vi "Create 3D Shapes.vi"(8 "error in (no error)":errorcluster, 11 "Frame Grabber Data In":T1={"Camera Session"="", "Frame"=refnum, "AVI Refnum"=refnum, "Codecs"=[], "Frame number"=0, "Tracking File Refnum"=refnum, "Tick Count"=0, "Probe Object"=refnum, "Playback Probe Data"=[], "Rigid Body"={"Position"={"x (mm)"=0.0, "y (mm)"=0.0, "z (mm)"=0.0}, "Orientation"={"Pitch (rad)"=0.0, "Yaw (rad)"=0.0, "Roll (rad)"=0.0}, "Quaternion"={"qx"=0.0, "qy"=0.0, "qz"=0.0, "qw"=0.0}, "Tracked?"=FALSE}, "Total no frames playback"=0, "Video FPS"=0.0, "Camera connected?"=FALSE, "Scene"=refnum, "Cropped Frame"=refnum, "Tracker FPS"=0.0, "Crop ROI"=[], "Presentation Values"=[], "Elapsed time (ms)"=0, "Camera frames playback"=0, "Refnums"={"Live Refnum"=refnum, "Record Refnum"=refnum, "Recording Settings Refnum"=refnum, "Playback Refnum"=refnum, "Frame Slider Refnum"=refnum, "Pause Refnum"=refnum, "Home Refnum"=refnum, "Crop Refnum"=refnum, "Clear Crop Refnum"=refnum, "stop refnum"=refnum, "Playback Rate Refnum"=refnum, "Operator Settings Refnums"=refnum, "Presentation Refnum"=refnum, "Gestation Refnum"=refnum, "Crop Time Frame Slider Refnum"=refnum, "Cancel Save Refnum"=refnum, "Reverse Playback Refnum"=refnum, "Connection Settings Refnum"=refnum}, "Dimensions"={"Probe Dimensions"={"Probe Width"=0.0, "Probe Depth"=1.0, "Probe Height"=0.0}, "Room Dimensions"={"Room Width"=0.0, "Room Depth"=0.0, "Room Height"=0.0}}, "Playback Data As Strings"=[], "Cropped Tracking File Refnum"=refnum, "Cropped AVI Refnum"=refnum, "Header"=[], "Total euclidian distance"=0.0, "Annotation File Path"=path "", "Playback File Path"=path ""}) -> (0 "error out":errorcluster={"status"=TRUE, "code"=1088, "source"="Property Node (arg 2) in NI_3D Picture Control.lvlib:Create Box.vi->Create 3D Shapes.vi->Init Frame Grabber.vi->Main.vi"}, 3 "Frame Grabber Data Out":T1={"Camera Session"="", "Frame"=refnum, "AVI Refnum"=refnum, "Codecs"=[], "Frame number"=0, "Tracking File Refnum"=refnum, "Tick Count"=0, "Probe Object"=refnum, "Playback Probe Data"=[], "Rigid Body"={"Position"={"x (mm)"=0.0, "y (mm)"=0.0, "z (mm)"=0.0}, "Orientation"={"Pitch (rad)"=0.0, "Yaw (rad)"=0.0, "Roll (rad)"=0.0}, "Quaternion"={"qx"=0.0, "qy"=0.0, "qz"=0.0, "qw"=0.0}, "Tracked?"=FALSE}, "Total no frames playback"=0, "Video FPS"=0.0, "Camera connected?"=FALSE, "Scene"=refnum, "Cropped Frame"=refnum, "Tracker FPS"=0.0, "Crop ROI"=[], "Presentation Values"=[], "Elapsed time (ms)"=0, "Camera frames playback"=0, "Refnums"={"Live Refnum"=refnum, "Record Refnum"=refnum, "Recording Settings Refnum"=refnum, "Playback Refnum"=refnum, "Frame Slider Refnum"=refnum, "Pause Refnum"=refnum, "Home Refnum"=refnum, "Crop Refnum"=refnum, "Clear Crop Refnum"=refnum, "stop refnum"=refnum, "Playback Rate Refnum"=refnum, "Operator Settings Refnums"=refnum, "Presentation Refnum"=refnum, "Gestation Refnum"=refnum, "Crop Time Frame Slider Refnum"=refnum, "Cancel Save Refnum"=refnum, "Reverse Playback Refnum"=refnum, "Connection Settings Refnum"=refnum}, "Dimensions"={"Probe Dimensions"={"Probe Width"=0.0, "Probe Depth"=1.0, "Probe Height"=0.0}, "Room Dimensions"={"Room Width"=0.0, "Room Depth"=0.0, "Room Height"=0.0}}, "Playback Data As Strings"=[], "Cropped Tracking File Refnum"=refnum, "Cropped AVI Refnum"=refnum, "Header"=[], "Total euclidian distance"=0.0, "Annotation File Path"=path "", "Playback File Path"=path ""})   [LabVIEW 2017]
uses:
  Controls/Frame Grabber Data.ctl
  <vilib>/userdefined/High Color/IMAQdx.ctl
  <vilib>/vision/Image Controls.llb/IMAQ Image.ctl
  <vilib>/vision/Avi.llb/IMAQ AVI2 Refnum.ctl
  Controls/Rigid Body Info.ctl
  Controls/Position.ctl
  Controls/Orientation.ctl
  Controls/Refnums.ctl
  Controls/Recording Settings.ctl
  Controls/Operator Settings.ctl
  Controls/Operator.ctl
  Controls/Connection Settings.ctl
  Controls/Tracker Type.ctl
  Controls/COM Port.ctl
  Controls/Dimensions.ctl
  Controls/Room Dimensions.ctl
  <vilib>/picture/3D Picture Control/Object/Create Object (name).vi
  <vilib>/picture/3D Picture Control/Object/Create Object (drawable).vi
  <vilib>/picture/3D Picture Control/Object/Add Object (no reference).vi
  <vilib>/picture/3D Picture Control/Object/Add Object (reference).vi
  <vilib>/picture/3D Picture Control/NI_3D Picture Control.lvlib
panel:
  out "Probe Object":refnum<vi>
  out "Scene":refnum<vi>(3d-picture)
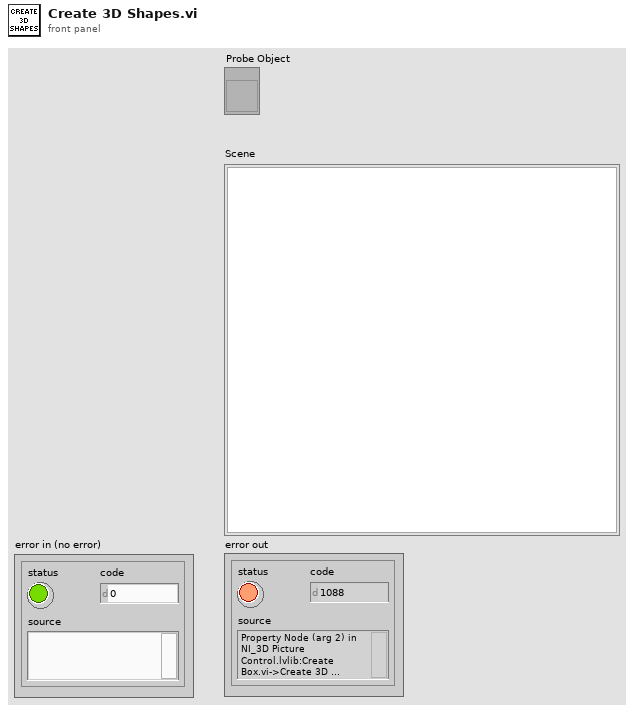
[diagram p1: front panel]
types:
  T1 = typedef "Frame Grabber Data.ctl" = cluster{"Camera Session":T2, "Frame":T3, "AVI Refnum":T4, "Codecs":string[], "Frame number":u32, "Tracking File Refnum":refnum<file>, "Tick Count":u32, "Probe Object":refnum<vi>, "Playback Probe Data":dbl[][], "Rigid Body":T5, "Total no frames playback":i32, "Video FPS":dbl, "Camera connected?":bool, "Scene":refnum<vi>, "Cropped Frame":T3, "Tracker FPS":dbl, "Crop ROI":i32[], "Presentation Values":string[], "Elapsed time (ms)":u32, "Camera frames playback":u32, "Refnums":T8, "Dimensions":T9, "Playback Data As Strings":string[][], "Cropped Tracking File Refnum":refnum<file>, "Cropped AVI Refnum":T4, "Header":string[], "Total euclidian distance":dbl, "Annotation File Path":path, "Playback File Path":path}
  T2 = typedef "IMAQdx.ctl" = refnum<k21>
  T3 = typedef "IMAQ Image.ctl" = refnum<image>
  T4 = typedef "IMAQ AVI2 Refnum.ctl" = refnum<k20>
  T5 = typedef "Rigid Body Info.ctl" = cluster{"Position":T6, "Orientation":T7, "Quaternion":cluster{"qx":sgl, "qy":sgl, "qz":sgl, "qw":sgl}, "Tracked?":bool}
  T6 = typedef "Position.ctl" = cluster{"x (mm)":sgl, "y (mm)":sgl, "z (mm)":sgl}
  T7 = typedef "Orientation.ctl" = cluster{"Pitch (rad)":sgl, "Yaw (rad)":sgl, "Roll (rad)":sgl}
  T8 = typedef "Refnums.ctl" = cluster{"Live Refnum":refnum<vi>, "Record Refnum":refnum<vi>, "Recording Settings Refnum":refnum<vi>, "Playback Refnum":refnum<vi>, "Frame Slider Refnum":refnum<vi>, "Pause Refnum":refnum<vi>, "Home Refnum":refnum<vi>, "Crop Refnum":refnum<vi>, "Clear Crop Refnum":refnum<vi>, "stop refnum":refnum<vi>, "Playback Rate Refnum":refnum<vi>, "Operator Settings Refnums":refnum<vi>, "Presentation Refnum":refnum<vi>, "Gestation Refnum":refnum<vi>, "Crop Time Frame Slider Refnum":refnum<vi>, "Cancel Save Refnum":refnum<vi>, "Reverse Playback Refnum":refnum<vi>, "Connection Settings Refnum":refnum<vi>}
  T9 = typedef "Dimensions.ctl" = cluster{"Probe Dimensions":cluster{"Probe Width":sgl, "Probe Depth":sgl, "Probe Height":sgl}, "Room Dimensions":T10}
  T10 = typedef "Room Dimensions.ctl" = cluster{"Room Width":dbl, "Room Depth":dbl, "Room Height":dbl}
  T11 = cluster{"Red":sgl, "Green":sgl, "Blue":sgl, "Alpha":sgl}
  T12 = enum16{"Inherit Value", "No Culling", "Cull Back Face", "Cull Front Face", "Cull Both Faces"}
  T13 = enum16{"Normal Bin", "Opaque Bin", "Transparent Bin"}
  T14 = cluster{"Probe Width":sgl, "Probe Depth":sgl, "Probe Height":sgl}
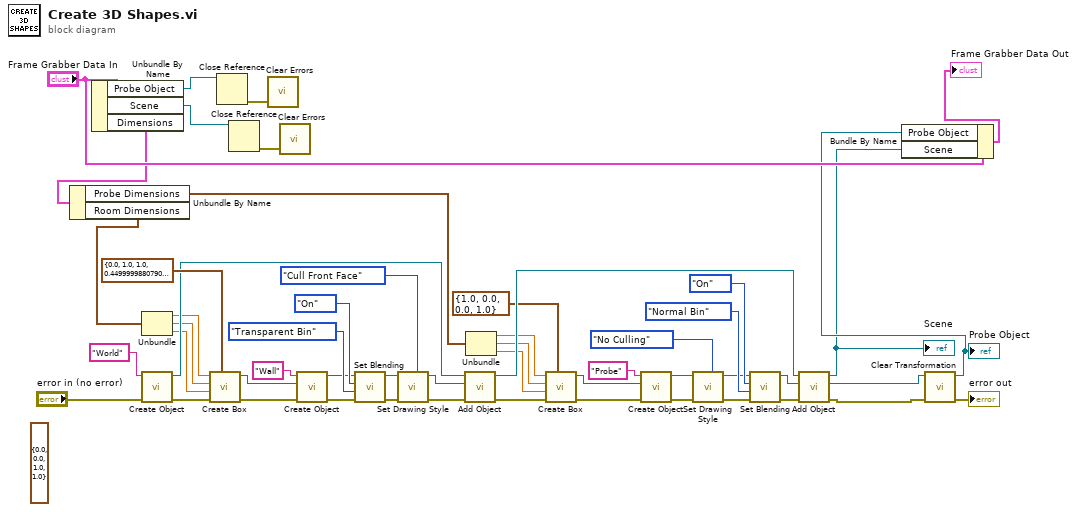
[diagram p0: block diagram]
diagram:
  (unwired) T11 {"Red"=0.0, "Green"=0.0, "Blue"=1.0, "Alpha"=1.0} ("Color")
  n1 = Unbundle By Name("Frame Grabber Data In") -> ("Probe Object"=w10:refnum<vi>, "Scene"=w9:refnum<vi>, "Dimensions"=w3:T9)
  n2 = Unbundle By Name(w3) -> ("Probe Dimensions"=w1:T14, "Room Dimensions"=w2:T10)
  n3 = Unbundle(w2) -> ("Room Width"=w20:dbl, "Room Depth"=w19:dbl, "Room Height"=w18:dbl)
  n4 = call-poly <vilib>:"Create Object.vi"("error in (no error)"="error in (no error)", "Name"="World") -> ("error out"=w50:errorcluster, "Scene:New Object"=w49:refnum<vi>)  [unwired: 8 in]
  n5 = call <vilib>:"Create Box.vi"("Color"=T11 {"Red"=0.0, "Green"=1.0, "Blue"=1.0, "Alpha"=0.45} ("Color 2"), "error in (no error)"=w50, "Length Z"=w18, "Length Y"=w19, "Length X"=w20) -> ("error out"=w48:errorcluster, "New Box Refnum"=w25:refnum<vi>)  [unwired: 5 in]
  n6 = Close Reference(reference=w10) -> (error out=w12:errorcluster)  [unwired: 1 in]
  n7 = Close Reference(reference=w9) -> (error out=w11:errorcluster)  [unwired: 1 in]
  n8 = call <vilib>:"Clear Errors.vi"("error in (no error)"=w12) -> ()  [unwired: 5 in, 2 out]
  n9 = call <vilib>:"Clear Errors.vi"("error in (no error)"=w11) -> ()  [unwired: 5 in, 2 out]
  n10 = call-poly <vilib>:"Create Object.vi"("error in (no error)"=w48, "Geometry"=w25, "Name"="Wall") -> ("error out"=w27:errorcluster, "Scene:New Object"=w28:refnum<vi>)  [unwired: 7 in]
  n11 = call <vilib>:"Set Blending.vi"("error in (no error)"=w27, "Bin"=T13."Transparent Bin", "Mode"=enum16{"Inherit Value", "Off", "On"}."On", "Scene Object In"=w28) -> ("error out"=w31:errorcluster, "Scene Object Out"=w32:refnum<vi>)  [unwired: 6 in]
  n12 = call <vilib>:"Set Drawing Style.vi"("Face Culling Mode"=T12."Cull Front Face" ("Draw Style:Face Culling Mode"), "error in (no error)"=w31, "Scene Object In"=w32) -> ("error out"=w43:errorcluster, "Scene Object Out"=w35:refnum<vi>)  [unwired: 7 in]
  n13 = call-poly <vilib>:"Add Object.vi"("error in (no error)"=w43, "New Object In"=w35, "Scene Object In"=w49) -> ("error out"=w51:errorcluster, "Scene Object Out"=w36:refnum<vi>)  [unwired: 7 in]
  n14 = Unbundle(w1) -> ("Probe Width"=w17:sgl, "Probe Depth"=w16:sgl, "Probe Height"=w15:sgl)
  n15 = call <vilib>:"Create Box.vi"("Color"=T11 {"Red"=1.0, "Green"=0.0, "Blue"=0.0, "Alpha"=1.0}, "error in (no error)"=w51, "Length Z"=w15, "Length Y"=w16, "Length X"=w17) -> ("error out"=w44:errorcluster, "New Box Refnum"=w26:refnum<vi>)  [unwired: 5 in]
  n16 = call-poly <vilib>:"Create Object.vi"("error in (no error)"=w44, "Geometry"=w26, "Name"="Probe") -> ("error out"=w45:errorcluster, "Scene:New Object"=w37:refnum<vi>)  [unwired: 7 in]
  n17 = call <vilib>:"Set Drawing Style.vi"("Face Culling Mode"=T12."No Culling", "error in (no error)"=w45, "Scene Object In"=w37) -> ("error out"=w46:errorcluster, "Scene Object Out"=w39:refnum<vi>)  [unwired: 7 in]
  n18 = call <vilib>:"Set Blending.vi"("error in (no error)"=w46, "Bin"=T13."Normal Bin" ("Blending:Bin"), "Mode"=enum16{"Inherit Value", "Off", "On"}."On", "Scene Object In"=w39) -> ("error out"=w47:errorcluster, "Scene Object Out"=w42:refnum<vi>)  [unwired: 6 in]
  n19 = call-poly <vilib>:"Add Object.vi"("error in (no error)"=w47, "New Object In"=w42, "Scene Object In"=w36) -> ("error out"=w4:errorcluster, "New Object Out"=w14:refnum<vi>, "Scene Object Out"=w5:refnum<vi>)  [unwired: 6 in]
  "Scene" <- w5
  n20 = call <vilib>:"Clear Transformation.vi"("error in (no error)"=w4, "Object Refnum In"=w14) -> ("error out"=→"error out":errorcluster, "Object Refnum Out"=w7:refnum<vi>)  [unwired: 8 in]
  "Probe Object" <- w7
  n21 = Bundle By Name(cluster="Frame Grabber Data In", "Probe Object"=w7, "Scene"=w5) -> (→"Frame Grabber Data Out":T1)
